vi "Resize Window and Reg VI.vi"(6 "Add Button Refnum":refnum<vi>, 8 "error in (no error)":errorcluster, 9 "Sub Panel Refnum":refnum<vi>, 10 "Actor Core Refnum":refnum<vi>, 11 "Form Window in":refnum<class "Form Window.lvclass">) -> (0 "error out":errorcluster, 3 "Form Window out":refnum<class "Form Window.lvclass">)   [LabVIEW 2020, in "Panel Form Controller.lvlib" / "Form Window.lvclass"]
uses:
  Form Window.lvclass
  C:/Users/User/Desktop/Raman Program/Database OOP/source/Forms AF/Form Controller/Panel Form Controller.lvclass
  C:/Program Files (x86)/National Instruments/LabVIEW 2020/vi.lib/MGI/Panel Manager/Panel Actor/Panel Actor/Panel Actor.lvclass
  Form Controller/Panel Form Controller.lvclass/Panel Form Controller.ctl
  <vilib>/MGI/Panel Manager/Panel/Panel/Subpanel/Subpanel.lvclass
  C:/Program Files (x86)/National Instruments/LabVIEW 2020/vi.lib/MGI/Panel Manager/Panel/Panel/Panel.lvclass
  <vilib>/MGI/Panel Manager/Panel/Panel/Subpanel/Subpanel.vi
  <vilib>/MGI/Panel Manager/Panel Actor/Panel Actor/Panel Actor.lvclass
  <vilib>/MGI/Panel Manager/Panel/Panel.lvlib
  Form Controller/Panel Form Controller.lvclass
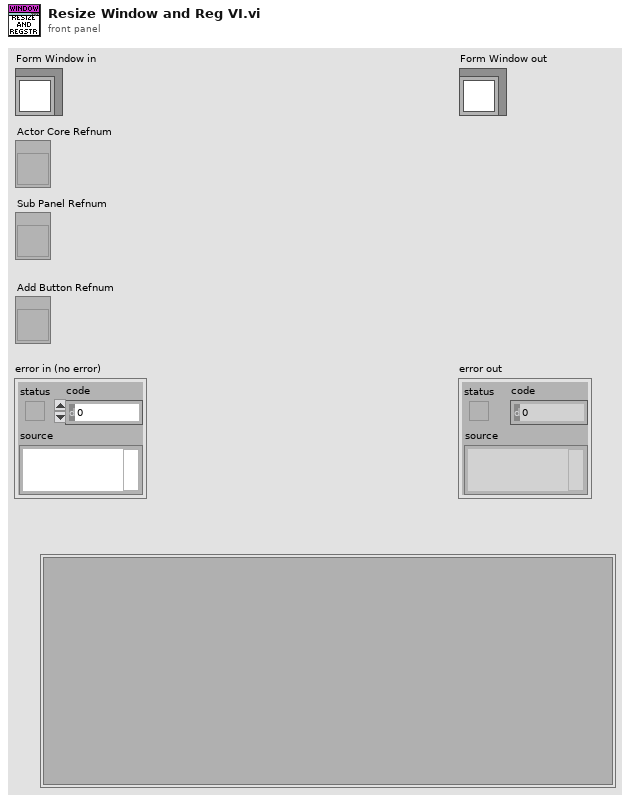
[diagram p1: front panel]
types:
  T1 = typedef "LVPointTypeDef.ctl" = cluster{"Horizontal":i16, "Vertical":i16}
  T2 = typedef "LVPositionTypeDef.ctl" = cluster{"Left":i32, "Top":i32}
  T3 = typedef "LVRectTypeDef.ctl" = cluster{"Left":i16, "Top":i16, "Right":i16, "Bottom":i16}
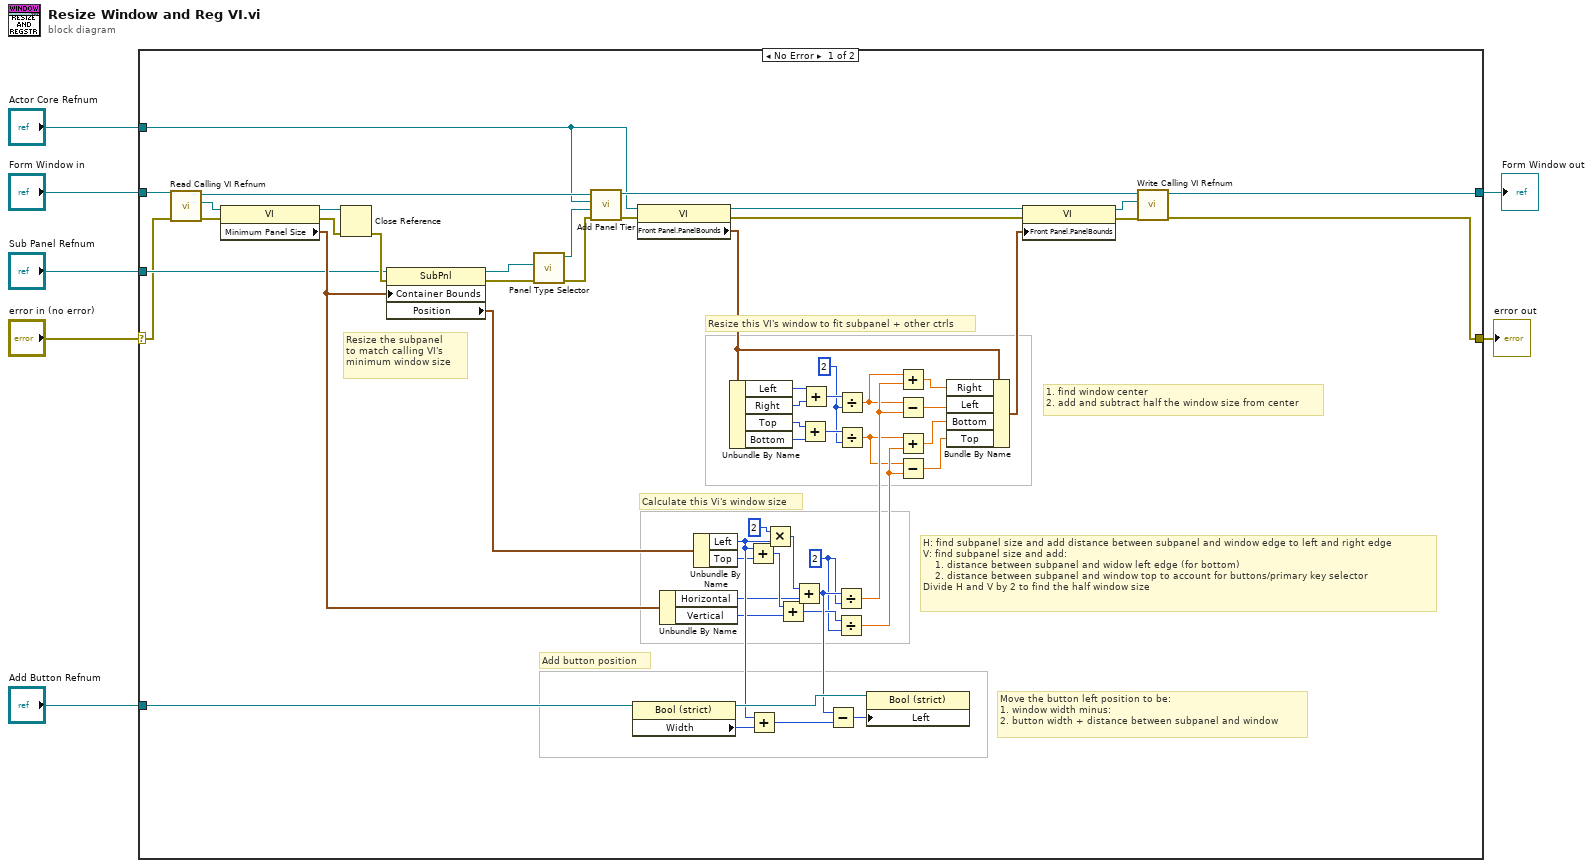
[diagram p0: block diagram]
diagram:
  n1 = case shown="No Error" "error in (no error)" {
    selector: "error in (no error)" -> [w9 w65]
    tunnel: [w10 w65] -> w6
    tunnel: [w15 w64] -> w4
    tunnel: "Form Window in" -> [w16 w64]
    tunnel: "Add Button Refnum" -> [w14 _]
    tunnel: "Sub Panel Refnum" -> [w13 _]
    tunnel: "Actor Core Refnum" -> [w8 _]
    frame No Error {
      w19 = 2
      w18 = 2
      # "Resize the subpanel\nto match calling VI's\nminimum window size"
      # "Move the button left position to be:\n1. window width minus:\n2. button width + distance between subpanel and window"
      # "H: find subpanel size and add distance between subpanel and window edge to left and right edge\nV: find subpanel size and add:\n    1. distance between subpanel and widow left edge (for bottom)\n    2. distance between subpanel and window top to account for buttons/primary key selector\nDivide H and V by 2 to find the half window size"
      # "1. find window center\n2. add and subtract half the window size from center"
      # "Resize this VI's window to fit subpanel + other ctrls"
      # "Calculate this Vi's window size"
      # "Add button position"
      n2 = call "Read Calling VI Refnum.vi"("error in (no error)"=w9, "Panel Form Controller in"=w16) -> ("error out"=w24:errorcluster, "Calling VI Refnum"=w21:refnum<vi>, "Panel Form Controller out"=w29:refnum<class "Form Window.lvclass">)  [unwired: 7 in]
      n3 = property class="VI"(reference=w21, error in=w24) -> (reference out=w26:refnum<vi>, error out=w27:errorcluster, "Minimum Panel Size"=w38:T1)
      n4 = Close Reference(reference=w26, error in (no error)=w27) -> (error out=w28:errorcluster)
      n5 = property class="SubPnl"(reference=w13, error in=w28, "Container Bounds"=w38) -> (reference out=w25:refnum<vi>, error out=w22:errorcluster, "Position"=w32:T2)
      n6 = call-poly <vilib>:"Panel Type Selector.vi"("Error In"=w22, "Sub Panel"=w25) -> ("Error Out"=w23:errorcluster, "Subpanel Out"=w20:refnum<class "Subpanel.lvclass">)  [unwired: 8 in]
      n7 = call <vilib>:"Add Panel Tier.vi"("Error In"=w23, "Old VI's Destination"=w20, "New VI Ref"=w8, "Panel Actor in"=w29) -> ("Error Out"=w31:errorcluster, "Panel Actor out"=w30:refnum<class "Form Window.lvclass">)  [unwired: 6 in]
      n8 = property class="Bool (strict)"(reference=w14) -> (reference out=w62:refnum<vi>, "Width"=w58:u32)  [unwired: 1 in, 1 out]
      n9 = property class="VI"(reference=w8, error in=w31) -> (reference out=w39:refnum<vi>, error out=w12:errorcluster, "Front Panel.PanelBounds"=w51:T3)
      n10 = Unbundle By Name(w38) -> ("Horizontal"=w34:i16, "Vertical"=w36:i16)
      n11 = Unbundle By Name(w32) -> ("Left"=w59:i32, "Top"=w35:i32)
      n12 = Unbundle By Name(w51) -> ("Left"=w41:i16, "Right"=w42:i16, "Top"=w43:i16, "Bottom"=w40:i16)
      n13 = Add(x=w59, y=w35) -> (x+y=w37:i32)
      n14 = Add(x=w59, y=w58) -> (x+y=w61:u32)
      n15 = Multiply(x=2, y=w59) -> (x*y=w33:i32)
      n16 = Add(x=w37, y=w36) -> (x+y=w46:i32)
      n17 = Add(x=w33, y=w34) -> (x+y=w60:i32)
      n18 = Add(x=w43, y=w40) -> (x+y=w45:i16)
      n19 = Add(x=w41, y=w42) -> (x+y=w44:i16)
      n20 = Subtract(x=w60, y=w61) -> (x-y=w63:u32)
      n21 = Divide(x=w60, y=w19) -> (x/y=w49:dbl)
      n22 = Divide(x=w46, y=w19) -> (x/y=w50:dbl)
      n23 = Divide(x=w44, y=w18) -> (x/y=w47:dbl)
      n24 = Divide(x=w45, y=w18) -> (x/y=w48:dbl)
      n25 = property class="Bool (strict)"(reference=w62, "Left"=w63) -> ()  [unwired: 1 in, 2 out]
      n26 = Add(x=w47, y=w49) -> (x+y=w52:dbl)
      n27 = Subtract(x=w47, y=w49) -> (x-y=w53:dbl)
      n28 = Add(x=w48, y=w50) -> (x+y=w54:dbl)
      n29 = Subtract(x=w48, y=w50) -> (x-y=w55:dbl)
      n30 = Bundle By Name(cluster=w51, "Right"=w52, "Left"=w53, "Bottom"=w54, "Top"=w55) -> (w56:T3)
      n31 = property class="VI"(reference=w39, error in=w12, "Front Panel.PanelBounds"=w56) -> (reference out=w57:refnum<vi>, error out=w11:errorcluster)
      n32 = call "Write Calling VI Refnum.vi"("error in (no error)"=w11, "Calling VI Refnum"=w57, "Panel Form Controller in"=w30) -> ("error out"=w10:errorcluster, "Panel Form Controller out"=w15:refnum<class "Form Window.lvclass">)  [unwired: 7 in]
    }
    frame Error {
    }
  }
  "error out" <- w6
  "Form Window out" <- w4
